vi "MALTCON get fixture reference.vi"() -> ()   [LabVIEW 2018]
uses:
  <instrlib>/AltonTech MALT/AltonTech MALT200817.lvlib
panel:
  out "Fixture Reference":string
  in  "Address":i32
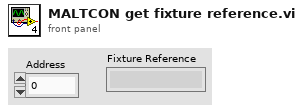
[diagram p1: front panel]
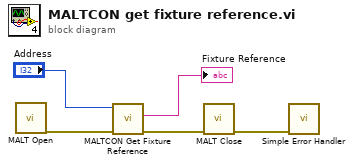
[diagram p0: block diagram]
diagram:
  n1 = call <instrlib>:"MALT Open.vi"() -> ("error out"=w5:errorcluster)  [unwired: 10 in, 1 out]
  n2 = call <instrlib>:"MALTCON Get Fixture Reference.vi"("error in"=w5, "Address"="Address") -> ("error out"=w2:errorcluster, "Value"=→"Fixture Reference":string)  [unwired: 7 in, 1 out]
  n3 = call <instrlib>:"MALT Close.vi"("error in"=w2) -> ("error out"=w1:errorcluster)  [unwired: 10 in]
  n4 = call <vilib>:"Simple Error Handler.vi"("error in (no error)"=w1) -> ()  [unwired: 4 in, 5 out]
